vi "create log folder.vi"(8 "error in (no error)":errorcluster, 11 "Log File in":refnum<class "Log File.lvclass">) -> (0 "error out":errorcluster, 3 "Log File out":refnum<class "Log File.lvclass">)   [LabVIEW 2018, in "Log File.lvclass"]
uses:
  Log File.lvclass
  Log File.lvclass/Log File.ctl
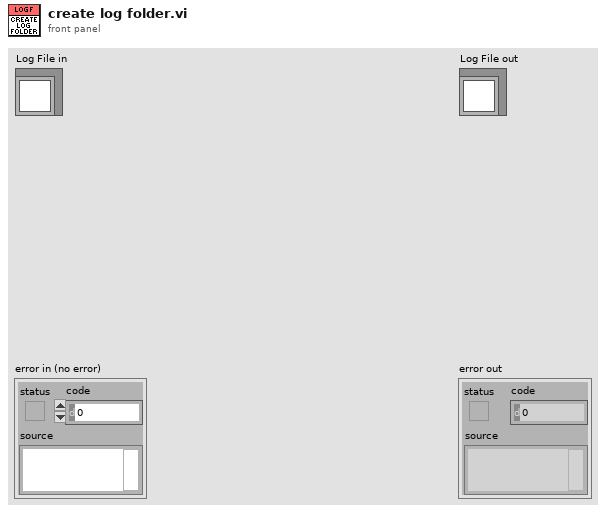
[diagram p1: front panel]
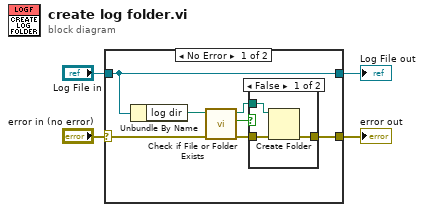
[diagram p0: block diagram]
diagram:
  n1 = case shown="No Error" "error in (no error)" {
    selector: "error in (no error)" -> [w9 w17]
    tunnel: [w10 w17] -> w3
    tunnel: [w11 w16] -> w1
    tunnel: "Log File in" -> [w11 w16]
    frame No Error {
      n2 = Unbundle By Name(w11) -> ("log dir"=w7:path)
      n3 = call <vilib>:"Check if File or Folder Exists.vi"("error in (no error)"=w9, "path"=w7) -> ("error out"=w8:errorcluster, "file or folder exists?"=w5:bool, "dup path"=w6:path)  [unwired: 7 in]
      n4 = case shown="False" w5 {
        tunnel: [w14 w15] -> w10
        tunnel: w8 -> [w13 w15]
        tunnel: w6 -> [w12 _]
        frame False {
          n5 = Create Folder(path (use dialog)=w12, error in=w13) -> (error out=w14:errorcluster)  [unwired: 1 in, 2 out]
        }
        frame True {
        }
      }
    }
    frame Error {
    }
  }
  "error out" <- w3
  "Log File out" <- w1
